vi "yokogawa.vi"   [LabVIEW 2011]
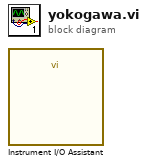
[diagram p0: block diagram]
diagram:
  n1 = call "Instrument I/O Assistant"() -> ()  [unwired: 25 in, 3 out]
